vi "MISC Decode Non Displayable Characters.vi"(0 "Input String":string, 11 "Error In (no error)":errorcluster) -> (4 "Output String":string, 15 "Error Out":errorcluster)   [LabVIEW 2011]
doc: "This routine replaces all non-displayable ASCII charactars with the corresponding Hex-ASCII representation of the character."
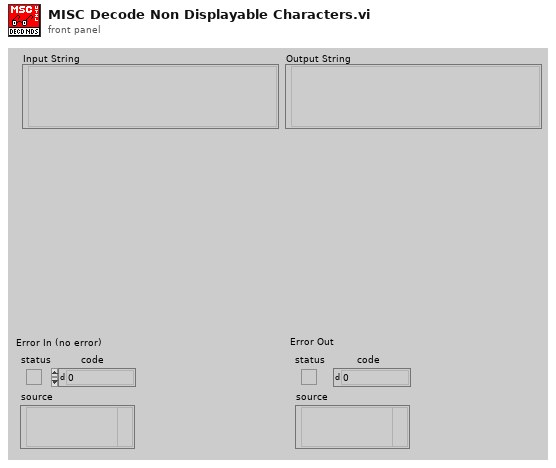
[diagram p1: front panel]
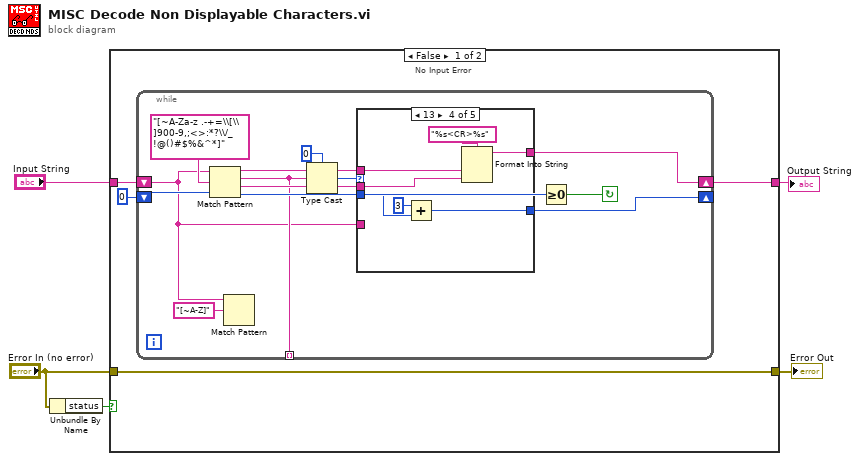
[diagram p0: block diagram]
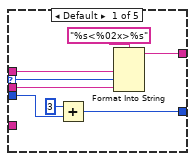
[diagram p2: hidden frame]
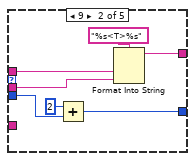
[diagram p3: hidden frame]
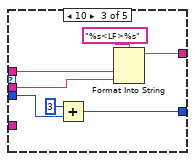
[diagram p4: hidden frame]
diagram:
  n1 = Unbundle By Name("Error In (no error)") -> ("status"=w5:bool)
  n2 = case shown="False" w5 {
    tunnel: [w9 w55] -> w4
    tunnel: "Error In (no error)" -> [w9 w55]
    tunnel: "Input String" -> [w8 w54]
    tunnel: [w6 w54] -> w1
    frame False {
      # "No Input Error"
      n3 = while {
        shift-left: 0 -> [w22]
        shift-right: [w18] -> _
        shift-left: w8 -> [w11]
        shift-right: [w14] -> w6
        tunnel: [w13] -> _ mode=indexing
        stop <- w17 continue-if-true
        n4 = Match Pattern(string=w11, regular expression="[~A-Za-z .-+=\\[\\]900-9,;<>:*?\\/_!@()#$%&^*]", offset (0)=w22) -> (before substring=w21:string, match substring=w13:string, after substring=w20:string, offset past match=w19:i32)
        n5 = Match Pattern(string=w11, regular expression="[~A-Z]") -> ()  [unwired: 5 out]
        n6 = Type Cast(type=u8 0, x=w13) -> (*(type *) &x=w16:u8)
        n7 = case shown="13" w16 {
          selector: w16 -> [w23 _ _ _ _]
          tunnel: w21 -> [w29 w36 w43 w50 _]
          tunnel: w20 -> [w28 w35 w42 w49 _]
          tunnel: w19 -> [w27 w34 w41 w48 w53]
          tunnel: [w26 w33 w40 w47 w52] -> w14
          tunnel: [w24 w31 w38 w45 w53] -> w18
          tunnel: w11 -> [_ _ _ _ w52]
          frame Default {
            n8 = Add(x=3, y=w27) -> (x+y=w24:i32)
            n9 = Format Into String(format string="%s<%02x>%s" ("Format String"), w29, w23, w28) -> (resulting string=w26:string)  [unwired: 2 in, 1 out]
          }
          frame 9 {
            n10 = Add(x=2, y=w34) -> (x+y=w31:i32)
            n11 = Format Into String(format string="%s<T>%s" ("Format String"), w36, w35) -> (resulting string=w33:string)  [unwired: 2 in, 1 out]
          }
          frame 10 {
            n12 = Add(x=3, y=w41) -> (x+y=w38:i32)
            n13 = Format Into String(format string="%s<LF>%s" ("Format String"), w43, w42) -> (resulting string=w40:string)  [unwired: 2 in, 1 out]
          }
          frame 13 {
            n14 = Add(x=3, y=w48) -> (x+y=w45:i32)
            n15 = Format Into String(format string="%s<CR>%s" ("Format String"), w50, w49) -> (resulting string=w47:string)  [unwired: 2 in, 1 out]
          }
          frame 0 {
          }
        }
        n16 = Greater Or Equal To 0?(x=w19) -> (x >= 0?=w17:bool)
      }
    }
    frame True {
      # "Input Error"
    }
  }
  "Error Out" <- w4
  "Output String" <- w1
